vi "Auto_PID_Drive.vi"(0 "Power":dbl, 1 "dt (s)":dbl=10.0 format="%.3f", 5 "Turning":dbl, 7 "PID Gains":T1={"proportional gain (Kc)"=0.09, "integral time (Ti, min)"=0.9, "derivative time (Td, min)"=0.001}, 9 "Yaw":dbl=-13.119872265000097, 11 "Turning_Setpoint":dbl, 12 "Turning_PID_Enable":bool) -> (4 "Power":dbl, 6 "Turning":dbl)   [LabVIEW 2016]
uses:
  <vilib>/Rock Robotics/Network Tables/NT Read Number.vi
  <vilib>/Rock Robotics/Network Tables/NT Write Number.vi
  <vilib>/addons/control/pid/pid.llb/PID (DBL).vi
  <vilib>/addons/control/pid/NI_PID_pid.lvlib
panel:
  out "Error":dbl
  out "Waveform Chart 2":dbl(graph)
  out "Waveform Chart":cluster{"Turning_Setpoint":dbl, "Yaw":dbl}(graph)={"Turning_Setpoint"=0.0, "Yaw"=-13.119872265000097}
  # "1/24/17\nKc=0.015\nTi=5\nTd=0.0005\nTurns slowly, but well"
  # "Drive Straight Constants\nKc=0.09\nTi=0.9\nTd=0.001\nNot good for turning"
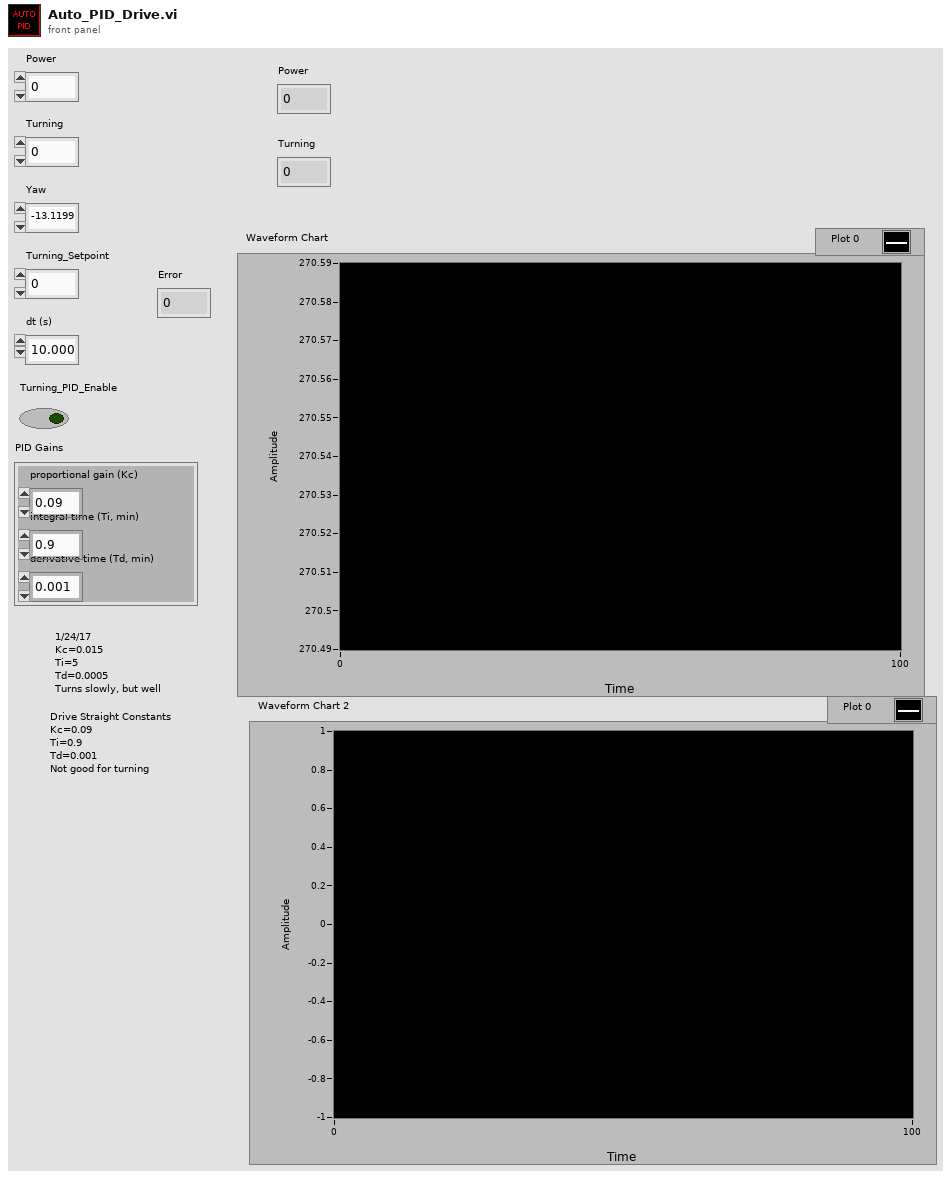
[diagram p1: front panel]
types:
  T1 = cluster{"proportional gain (Kc)":dbl, "integral time (Ti, min)":dbl, "derivative time (Td, min)":dbl}
  T2 = cluster{"Power":dbl, "Yaw":dbl, "Turning_PID_Enable":bool, "Turning":dbl, "Turning_Setpoint":dbl, "PID Gains":cluster{"proportional gain (Kc)":dbl, "integral time (Ti, min)":dbl, "derivative time (Td, min)":dbl}, "dt (s)":dbl}
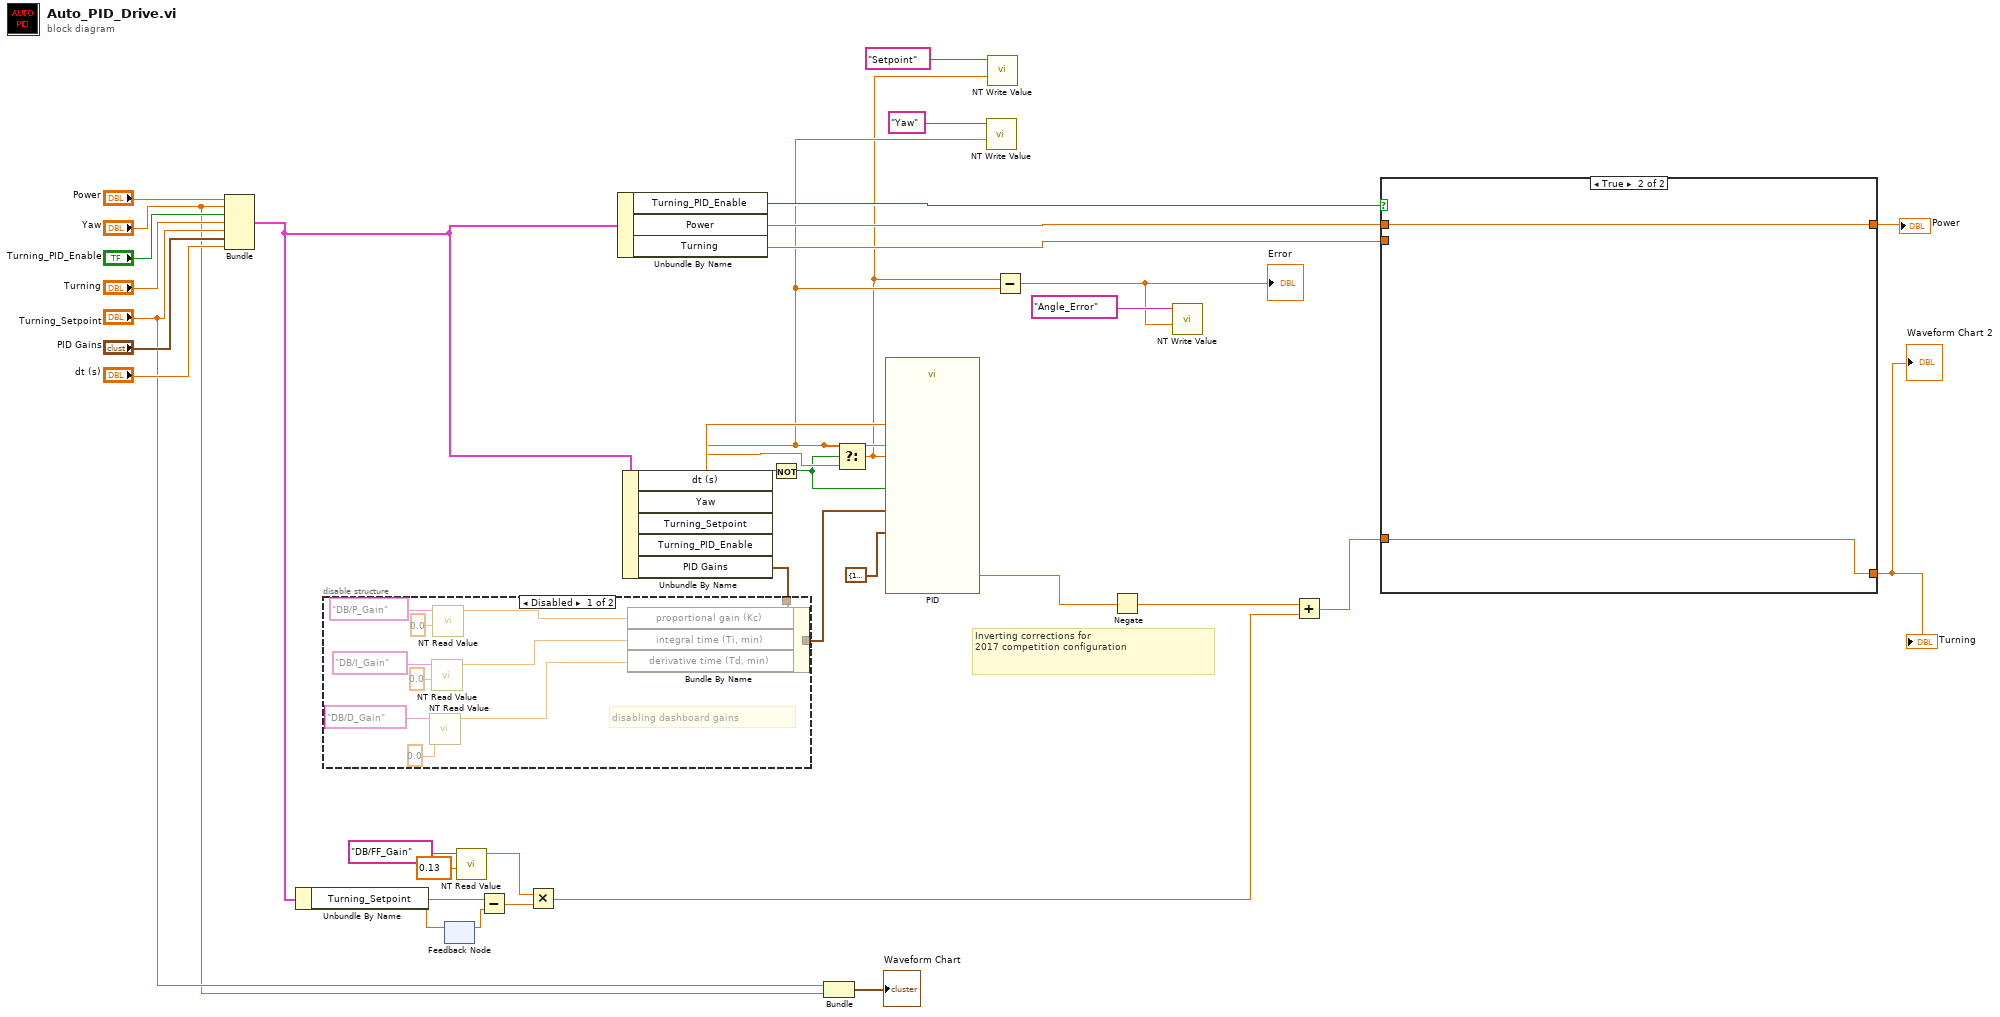
[diagram p0: block diagram]
diagram:
  # "Inverting corrections for\n2017 competition configuration"
  n1 = Bundle("Power"="Power", "Yaw"="Yaw", "Turning_PID_Enable"="Turning_PID_Enable", "Turning"="Turning", "Turning_Setpoint"="Turning_Setpoint", "PID Gains"="PID Gains", "dt (s)"="dt (s)") -> (w23:T2)  [unwired: 1 in]
  n2 = Unbundle By Name(w23) -> ("Turning_Setpoint"=w26:dbl)
  n3 = feedback-in #1(w26) -> ()
  n4 = feedback #1() -> (w25:dbl)  [unwired: 1 in]
  n5 = call-poly <vilib>:"NT Read Value.vi"("Default Value"=0.13, "Name"="DB/FF_Gain" ("refnum name")) -> ("Numeric"=w11:dbl)  [unwired: 8 in, 1 out]
  n6 = Subtract(x=w26, y=w25) -> (x-y=w24:dbl)
  n7 = Multiply(x=w11, y=w24) -> (x*y=w19:dbl)
  n8 = Unbundle By Name(w23) -> ("Turning_PID_Enable"=w22:bool, "Power"=w27:dbl, "Turning"=w33:dbl)
  n9 = Unbundle By Name(w23) -> ("dt (s)"=w18:dbl, "Yaw"=w6:dbl, "Turning_Setpoint"=w15:dbl, "Turning_PID_Enable"=w17:bool, "PID Gains"=w2:T1)
  n10 = disable-structure shown="Disabled" {
    disable-tunnel: [w47 w49] -> w3
    disable-tunnel: [w38 _] -> _
    disable-tunnel: w2 -> [w38 w49]
    frame Disabled {
      # "disabling dashboard gains"
      n11 = call-poly <vilib>:"NT Read Value.vi"("Default Value"=0.0, "Name"="DB/D_Gain" ("refnum name")) -> ("Numeric"=w40:dbl)  [unwired: 8 in, 1 out]
      n12 = call-poly <vilib>:"NT Read Value.vi"("Default Value"=0.0, "Name"="DB/I_Gain" ("refnum name")) -> ("Numeric"=w41:dbl)  [unwired: 8 in, 1 out]
      n13 = call-poly <vilib>:"NT Read Value.vi"("Default Value"=0.0, "Name"="DB/P_Gain" ("refnum name")) -> ("Numeric"=w42:dbl)  [unwired: 8 in, 1 out]
      n14 = Bundle By Name(cluster=w38, "proportional gain (Kc)"=w42, "integral time (Ti, min)"=w41, "derivative time (Td, min)"=w40) -> (w47:T1)
    }
    frame Enabled {
    }
  }
  n15 = Not(x=w17) -> (.not. x?=w14:bool)
  n16 = Bundle("Turning_Setpoint"="Turning_Setpoint", "Yaw"="Yaw") -> (→"Waveform Chart":cluster{"Turning_Setpoint":dbl, "Yaw":dbl})  [unwired: 1 in]
  n17 = Select(t=w6, s=w14, f=w15) -> (s? t:f=w5:dbl)
  n18 = call-poly <vilib>:"PID.vi"("reinitialize? (F)"=w14, "output range"=cluster{"output high":dbl, "output low":dbl} {"output high"=1.0, "output low"=-1.0}, "dt (s)"=w18, "PID gains"=w3, "process variable"=w6, "setpoint"=w5) -> ("output"=w4:dbl)  [unwired: 4 in, 1 out]
  n19 = call-poly <vilib>:"NT Write Value.vi"("Numeric"=w6, "Name"="Yaw") -> ()  [unwired: 9 in, 1 out]
  n20 = call-poly <vilib>:"NT Write Value.vi"("Numeric"=w5, "Name"="Setpoint") -> ()  [unwired: 9 in, 1 out]
  n21 = Subtract(x=w5, y=w6) -> (x-y=w9:dbl)
  "Error" <- w9
  n22 = Negate(x=w4) -> (-x=w1:dbl)
  n23 = call-poly <vilib>:"NT Write Value.vi"("Numeric"=w9, "Name"="Angle_Error") -> ()  [unwired: 9 in, 1 out]
  n24 = Add(x=w1, y=w19) -> (x+y=w16:dbl)
  n25 = case shown="True" w22 {
    tunnel: w27 -> [w51 w53]
    tunnel: w33 -> [w50 _]
    tunnel: [w51 w53] -> w32
    tunnel: [w50 w52] -> w21
    tunnel: w16 -> [_ w52]
    frame False {
    }
    frame True {
    }
  }
  "Power" <- w32
  "Turning" <- w21
  "Waveform Chart 2" <- w21
